vi "Single IO (depreciated).vi"() -> ()   [LabVIEW 2021]
panel:
  in  "x1":i32
  in  "Handle In":i32
  in  "IOType":u16(ring) items=["LJ_ioANALOG_INPUT", "LJ_ioANALOG_OUTPUT", "LJ_ioDIGITAL_BIT_IN", "LJ_ioDIGITAL_PORT_IN", "LJ_ioDIGITAL_BIT_OUT", "LJ_ioDIGITAL_PORT_OUT", "LJ_ioCOUNTER", "LJ_ioTIMER"]
  in  "error in":errorcluster
  out "error out":errorcluster
  in  "Value Write":dbl format="%.2f"
  out "Value Read":dbl format="%.6f"
  out "Handle Out":i32
  in  "Channel":i32
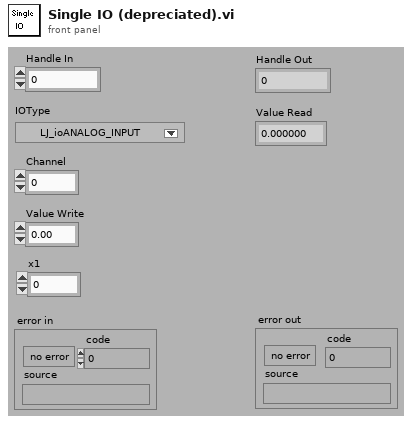
[diagram p1: front panel]
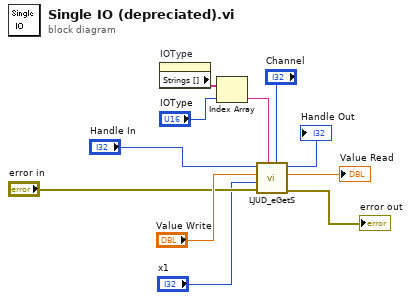
[diagram p0: block diagram]
diagram:
  n1 = property on="IOType" class="Ring (strict)"() -> ("Strings []"=w6:string[])  [unwired: 2 in, 2 out]
  n2 = Index Array(array=w6, index="IOType") -> (element=w4:string)
  n3 = call "LJUD_eGetS.vi"("Channel"="Channel", "IOType"=w4, "error in"="error in", "x1"="x1", "Value Write"="Value Write", "Handle In"="Handle In") -> ("error out"=→"error out":errorcluster, "Value Read"=→"Value Read":dbl, "Handle Out"=→"Handle Out":i32)  [unwired: 3 in]
